vi "Remove Unused Connections.vi"(11 "TCP slave in":refnum<class "TCP Slave.lvclass">) -> (0 "error out":errorcluster)   [LabVIEW 2017, in "SubVIs.lvlib" / "TCP Slave.lvclass"]
uses:
  <vilib>/Modbus/subvis/Protocol/TCP/TCP Slave/TCP Slave.lvclass
  <vilib>/Modbus/subvis/Protocol/TCP/TCP Slave/TCP Slave.lvclass/TCP Slave.ctl
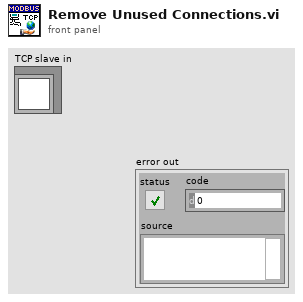
[diagram p1: front panel]
types:
  T1 = typedef "SubVIs.lvlib/TCP Slave.lvclass/Connection Counter.ctl" = cluster{"Currently Connected":u32, "Connection Records":refnum<data-value>[]}
  T2 = cluster{"Connected?":bool, "IP address":string, "connection error":errorcluster}
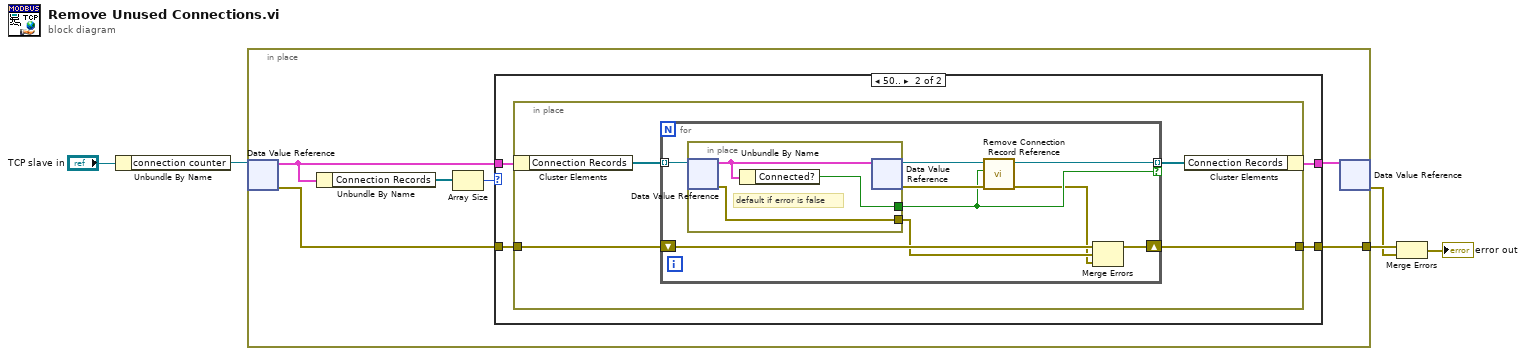
[diagram p0: block diagram]
diagram:
  n1 = Unbundle By Name("TCP slave in") -> ("connection counter"=w4:refnum<data-value>)
  n2 = in-place {
    in-place-border: [w6] -> w2
    n3 = in-place-dvr #1(w4) -> (w8:T1, w7:errorcluster)
    n4 = Unbundle By Name(w8) -> ("Connection Records"=w10:refnum<data-value>[])
    n5 = Array Size(array=w10) -> (size(s)=w11:i32)
    n6 = case shown="50.." w11 {
      tunnel: [w13 w16] -> w9
      tunnel: w8 -> [w13 w17]
      tunnel: w7 -> [w12 w15]
      tunnel: [w12 w14] -> w6
      frame Default {
      }
      frame 50.. {
        n7 = in-place {
          in-place-border: w15 -> [w19]
          in-place-border: [w18] -> w14
          n8 = in-place-cluster #2(w17) -> ("Connection Records"=w21:refnum<data-value>[])
          n9 = for {
            tunnel: w21 -> [w30] mode=indexing
            tunnel: [w25] -> w20 mode=indexing if=w23
            shift-right: [w29] -> w18
            shift-left: w19 -> [w28]
            n10 = in-place {
              in-place-border: [w32] -> w23
              in-place-border: [w31] -> w27
              # "default if error is false"
              n11 = in-place-dvr #3(w30) -> (w33:T2, w31:errorcluster)
              n12 = Unbundle By Name(w33) -> ("Connected?"=w32:bool)
              n13 = in-place-dvr #3(w33) -> (w26:refnum<data-value>, w24:errorcluster)
            }
            n14 = call <vilib>:"Remove Connection Record Reference.vi"("error in (no error)"=w24, "Connected?"=w23, "Data Value Reference in"=w26) -> ("error out"=w22:errorcluster, "Data Value Reference out"=w25:refnum<data-value>)  [unwired: 7 in]
            n15 = Merge Errors(w28, w27, w22) -> (w29:errorcluster)
          }
          n16 = in-place-cluster #2("Connection Records"=w20) -> (w16:T1)
        }
      }
    }
    n17 = in-place-dvr #1(w9) -> (w1:errorcluster)  [unwired: 1 out]
  }
  n18 = Merge Errors(w2, w1) -> (→"error out":errorcluster)
